vi "position process.vi"(8 "Error In":errorcluster, 11 "main-national data in":T1) -> (0 "Error Out":errorcluster, 3 "main-national data out":T1)   [LabVIEW 2019]
uses:
  ctl/main data-national.ctl
  ctl/position set.ctl
  ctl/position name.ctl
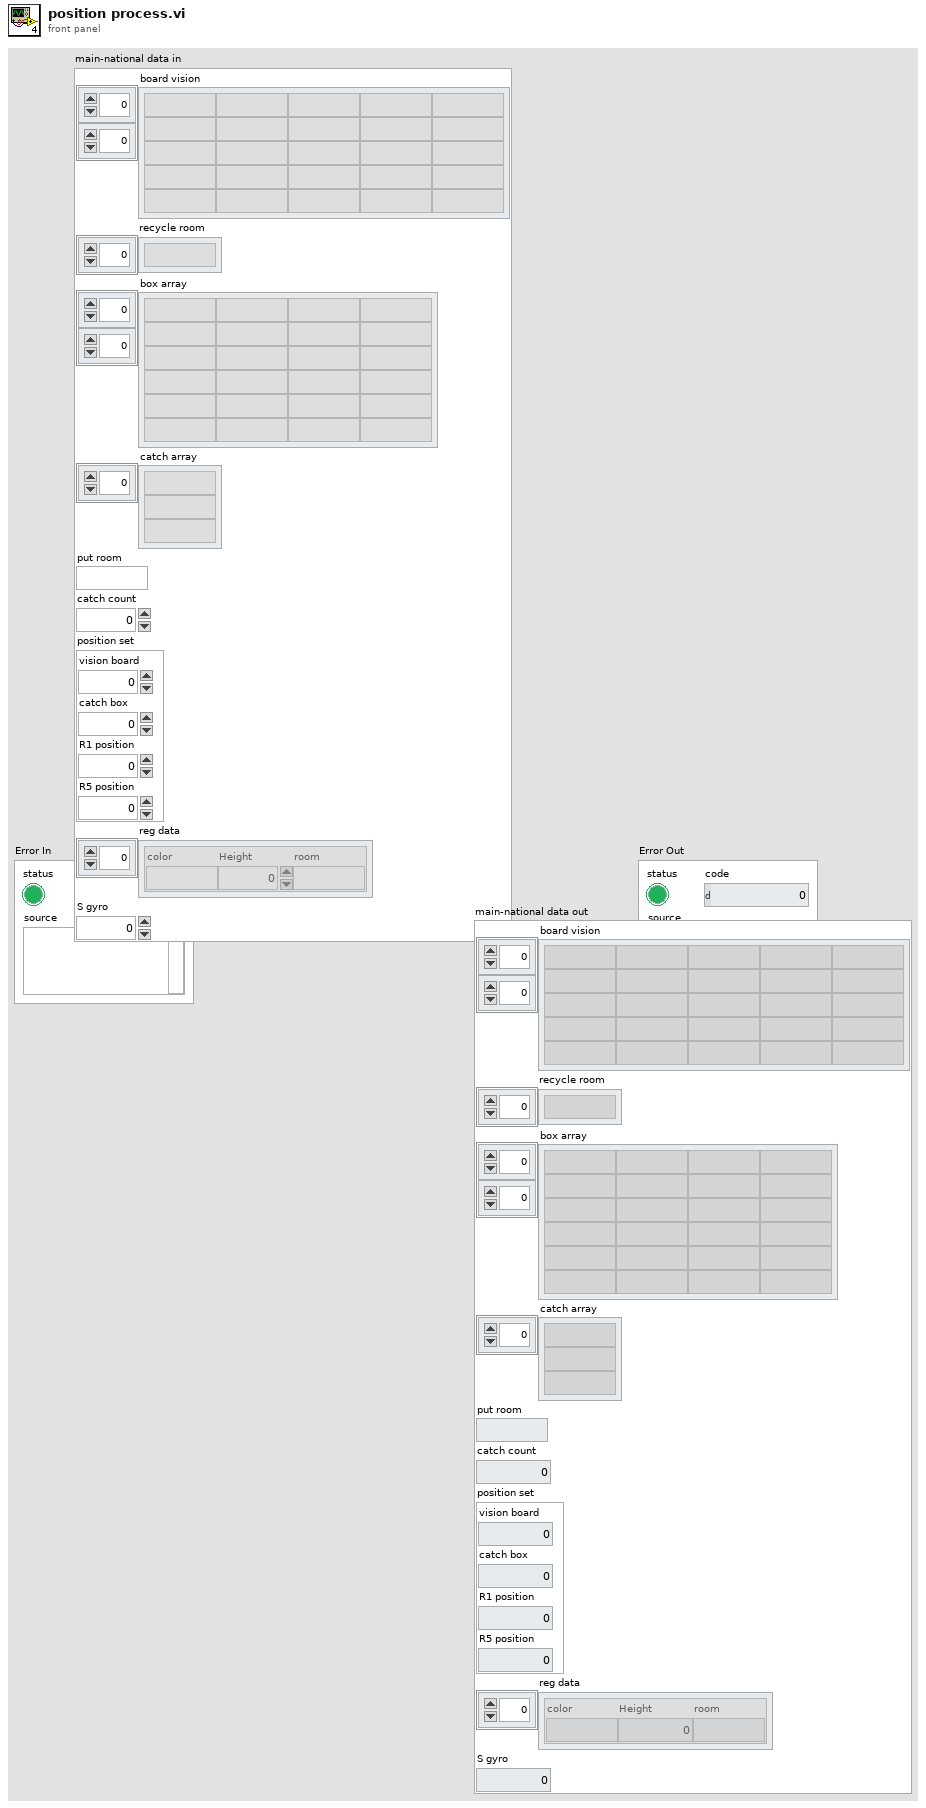
[diagram p1: front panel]
types:
  T1 = typedef "main data-national.ctl" = cluster{"board vision":string[][], "recycle room":string[], "box array":string[][], "catch array":string[], "put room":string, "catch count":dbl, "position set":T2, "reg data":cluster{"color":string, "Height":i32, "room":string}[], "S gyro":dbl}
  T2 = typedef "position set.ctl" = cluster{"vision board":dbl, "catch box":dbl, "R1 position":dbl, "R5 position":dbl}
  T3 = typedef "position name.ctl" = enum16{"S-zone", "out S", "vision board-vision", "out box", "box catch", "room center", "room right", "room left", "R2", "R4", "only rotate", "out recy", "recycle", "R3", "near board", "box poxition", "R1", "R5", "R1-d", "R5-d", "R3.4", "align center.1", "align center.5", "R2-d", "R2-r", "far center"}
  T4 = cluster{"vision board":dbl, "catch box":dbl, "R1 position":dbl, "R5 position":dbl}
  T5 = typedef "position array.ctl" = cluster{"position":T3, "X":dbl, "Y":dbl}
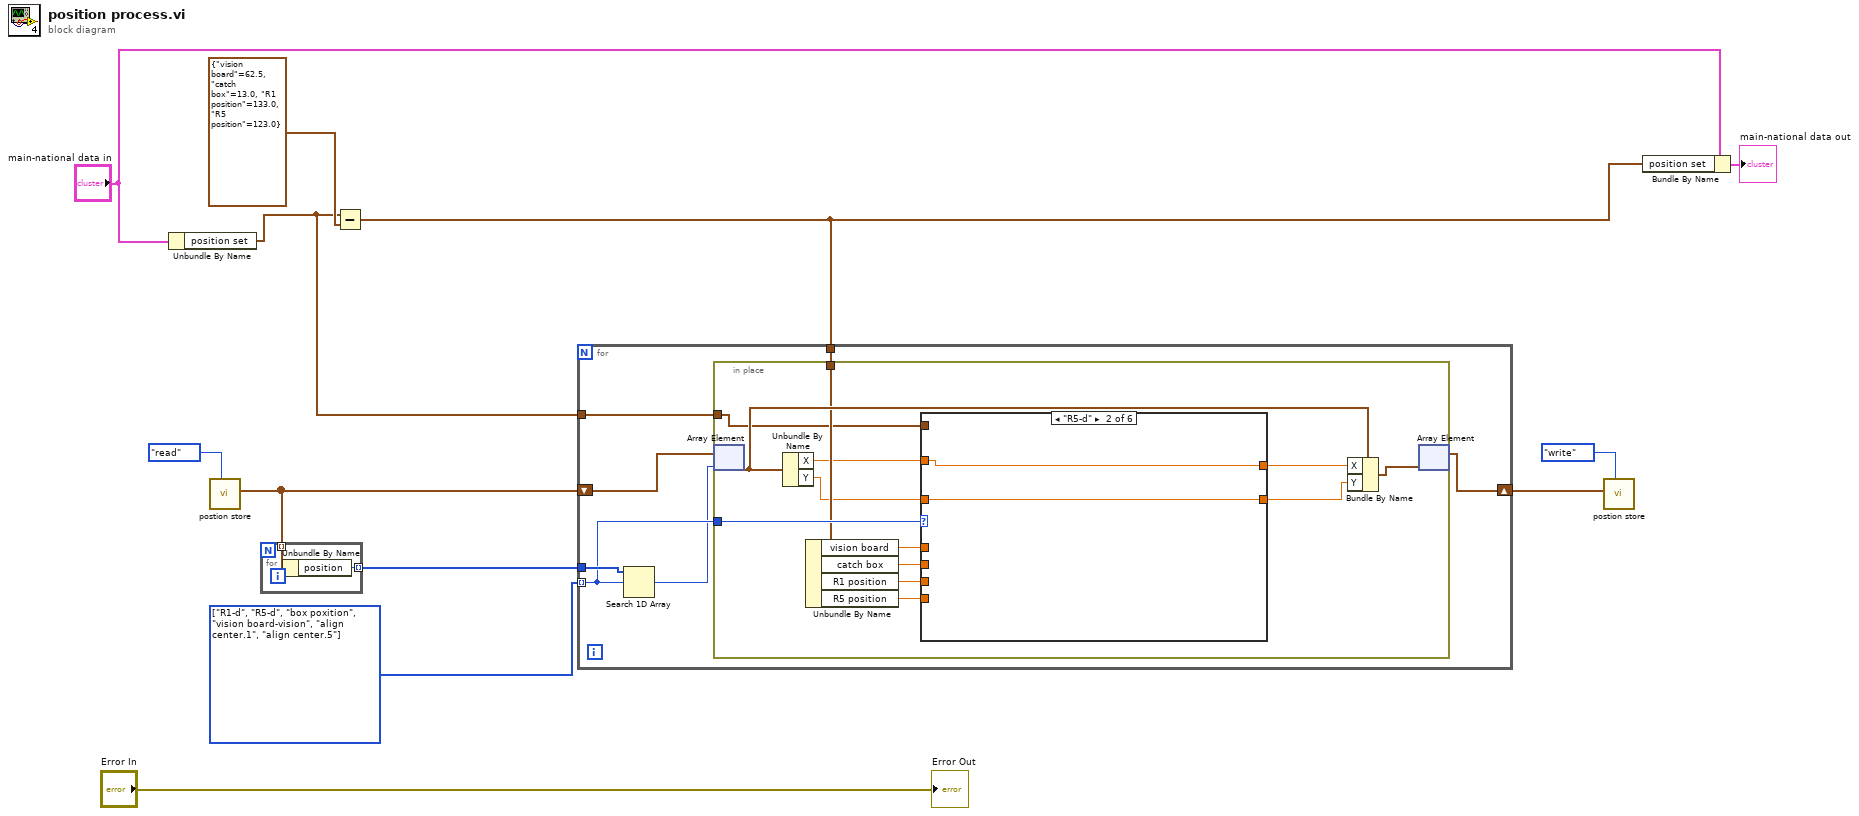
[diagram p0: block diagram]
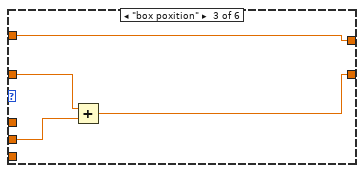
[diagram p3: hidden frame]
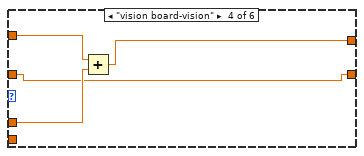
[diagram p4: hidden frame]
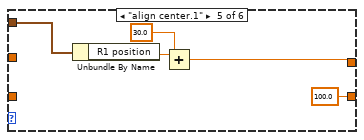
[diagram p5: hidden frame]
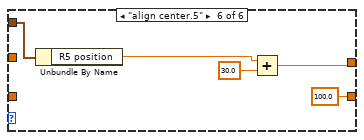
[diagram p6: hidden frame]
diagram:
  w5 = T3[] [enum."R1-d", enum."R5-d", enum."box poxition", enum."vision board-vision", enum."align center.1", enum."align center.5"] items=["S-zone", "out S", "vision board-vision", "out box", "box catch", "room center", "room right", "room left", "R2", "R4", "only rotate", "out recy", "recycle", "R3", "near board", "box poxition", "R1", "R5", "R1-d", "R5-d", "R3.4", "align center.1", "align center.5", "R2-d", "R2-r", "far center"] ("element")
  n1 = Unbundle By Name("main-national data in") -> ("position set"=w1:T2)
  n2 = call "postion store.vi"("R/W"=enum16{"write", "read"}."read") -> ("read"=w7:T5[])  [unwired: 10 in]
  n3 = for {
    tunnel: w7 -> [w14] mode=indexing
    tunnel: [w13] -> w6 mode=indexing
    n4 = Unbundle By Name(w14) -> ("position"=w13:T3)
  }
  n5 = Subtract(x=w1, y=T4 {"vision board"=62.5, "catch box"=13.0, "R1 position"=133.0, "R5 position"=123.0} ("position set")) -> (x-y=w4:T2)
  n6 = for {
    shift-right: [w16] -> w3
    shift-left: w7 -> [w19]
    tunnel: w6 -> [w21]
    tunnel: w5 -> [w20] mode=indexing
    tunnel: w4 -> [w17]
    tunnel: w1 -> [w15]
    n7 = Search 1D Array(1D array=w21, element=w20) -> (index of element=w18:i32)  [unwired: 1 in]
    n8 = in-place {
      in-place-border: w20 -> [w34]
      in-place-border: w17 -> [w32]
      in-place-border: w15 -> [w22]
      n9 = in-place-array #1(w19, w18) -> (w33:T5)
      n10 = Unbundle By Name(w33) -> ("X"=w31:dbl, "Y"=w27:dbl)
      n11 = Unbundle By Name(w32) -> ("vision board"=w24:dbl, "catch box"=w25:dbl, "R1 position"=w30:dbl, "R5 position"=w26:dbl)
      n12 = case shown="\"R5-d\"" w34 {
        tunnel: w31 -> [w36 w38 w39 w46 _ _]
        tunnel: w30 -> [_ _ _ _ _ _]
        tunnel: [w36 w38 w39 w44 w48 w53] -> w29
        tunnel: [w35 w37 w40 w43 100.0 ("Y") 100.0 ("Y")] -> w28
        tunnel: w27 -> [w35 w37 w42 w43 _ _]
        tunnel: w26 -> [_ _ _ _ _ _]
        tunnel: w25 -> [_ _ w41 _ _ _]
        tunnel: w24 -> [_ _ _ w45 _ _]
        tunnel: w22 -> [_ _ _ _ w51 w56]
        frame "R1-d", Default {
        }
        frame "R5-d" {
        }
        frame "box poxition" {
          n13 = Add(x=w42, y=w41) -> (x+y=w40:dbl)
        }
        frame "vision board-vision" {
          n14 = Add(x=w46, y=w45) -> (x+y=w44:dbl)
        }
        frame "align center.1" {
          n15 = Unbundle By Name(w51) -> ("R1 position"=w50:dbl)
          n16 = Add(x=w50, y=30.0) -> (x+y=w48:dbl)
        }
        frame "align center.5" {
          n17 = Unbundle By Name(w56) -> ("R5 position"=w55:dbl)
          n18 = Add(x=w55, y=30.0) -> (x+y=w53:dbl)
        }
      }
      n19 = Bundle By Name(cluster=w33, "X"=w29, "Y"=w28) -> (w23:T5)
      n20 = in-place-array #1(w23) -> (w16:T5[])  [unwired: 1 out]
    }
  }
  n21 = call "postion store.vi"("R/W"=enum16{"write", "read"}."write", "Write"=w3) -> ()  [unwired: 9 in, 1 out]
  n22 = Bundle By Name(cluster="main-national data in", "position set"=w4) -> (→"main-national data out":T1)
  "Error Out" <- "Error In"
